vi "Write or Update data Database.vi"(8 "error in (no error)":errorcluster caption="entrée d'erreur (pas d'erreur)", 10 "Function":enum16{"Set Data", "Update Data"}(ring), 11 "Sequencer IN":refnum<class "Sequencer_With_Database.lvclass">) -> (0 "error out":errorcluster caption="sortie d'erreur", 3 "Sequencer Out":refnum<class "Sequencer_With_Database.lvclass">)   [LabVIEW 2020, in "Library Core.lvlib" / "Sequencer_With_Database.lvclass"]
uses:
  Sequencer_With_Database.lvclass
  C:/Users/ngarcin/OneDrive - Altyor/Standard TB/Suite TB45/Class/Sequencer/Sequencer (Default)/Sequencer (Default).lvclass
  Commun VI/TypeDef/Variable Printable.ctl
  Database/Database Altyor/Database Altyor.lvclass
  C:/Users/ngarcin/OneDrive - Altyor/Standard TB/Suite TB45/Class/Database/Database drivers/Database Drivers.lvclass
  JSON API/JSON Value/Set from JSON string.vi
  JSON API/Variant JSON/Variant to JSON.vi
  JSON API/JSON Value/Get Item by name array.vi
  Instrument/Instrument (Default)/Class Instrument (Default).lvclass
  JSON API/JSON Value/JSON Value.lvclass
  Commun VI/Library Commun.lvlib
  JSON API/Variant JSON/Variant JSON.lvlib
  JSON API/Get Polymorphic/JSON GetSet.lvlib
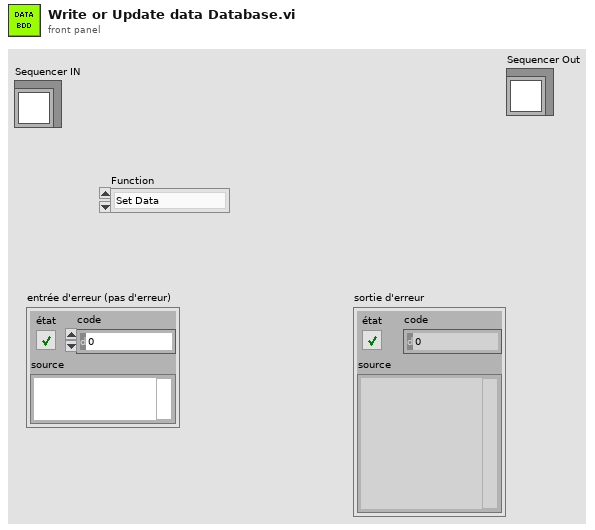
[diagram p1: front panel]
types:
  T1 = cluster{"Connection Name ODBC":string, "DatabaseName":string, "Condition":string, "Type Data ":enum16{"Data Product", "Data Test"}, "Database Altyor":refnum<class "Database Altyor.lvclass">}
  T2 = typedef "Variable Printable.ctl" = string
  T3 = enum16{"Get Variable", "Get All Variables", "Set Variable", "Delete Variable", "Delete All Variable"}
  T4 = cluster{"idTest":u32, "CreationDate":string, "EndOfProduction":string, "OrderNumber":string, "Batch":string, "ProductName":string, "PartNumber":string, "SerialNumber":string, "Operator":string, "Result":string, "AdditionalInformation":string}
  T5 = cluster{"idTest":u32, "CreationDate":string, "EndOfProduction":string, "OrderNumber":string, "Batch":string, "ProductName":string, "PartNumber":string, "SerialNumber":string, "Operator":string, "Result":string, "AdditionalInformation":string}[]
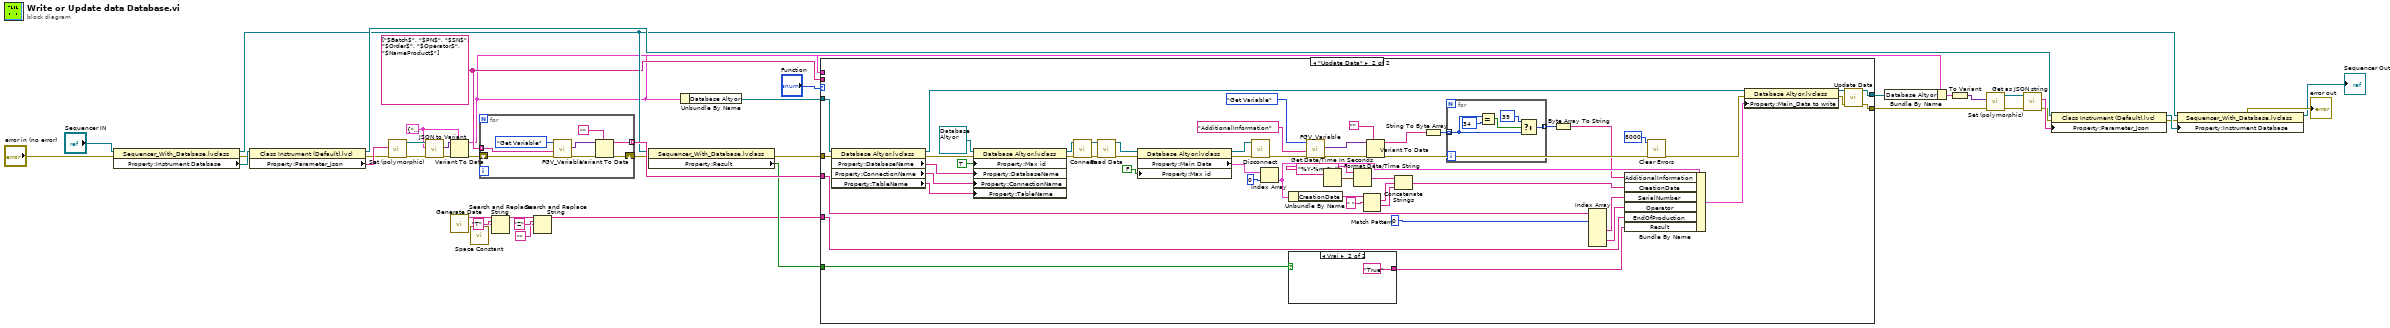
[diagram p0: block diagram]
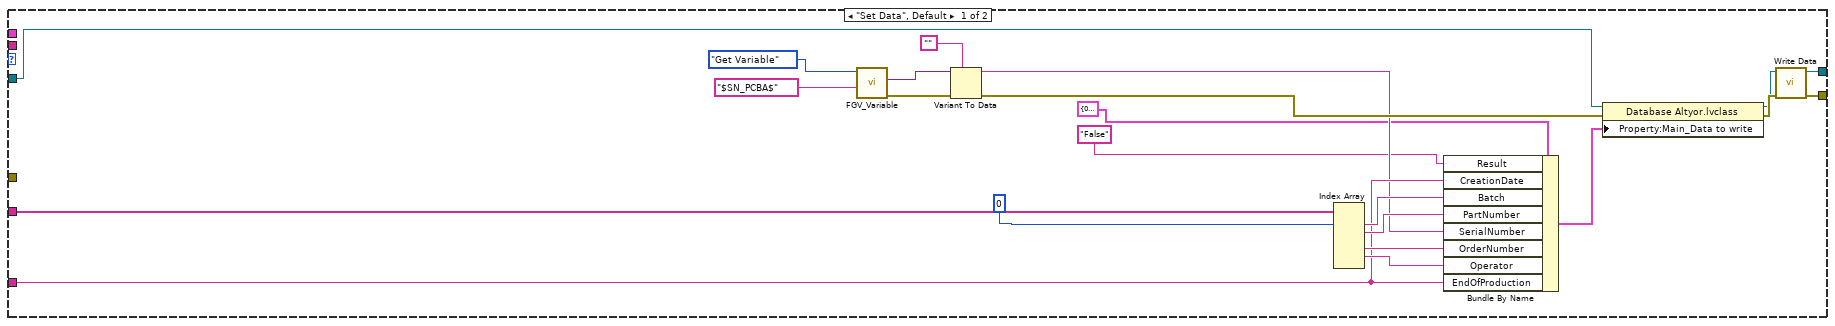
[diagram p2: hidden frame]
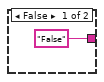
[diagram p3: hidden frame]
diagram:
  w9 = T1 {"Connection Name ODBC"="", "DatabaseName"="", "Condition"="", "Type Data "=enum."Data Product", "Database Altyor"=refnum} ("Parameter")
  w12 = T2[] ["$Batch$", "$PN$", "$SN$", "$Order$", "$Operator$", "$NameProduct$"]
  n1 = property class="Sequencer_With_Database.lvclass"(reference="Sequencer IN", error in="error in (no error)") -> (reference out=w14:refnum<class "Sequencer_With_Database.lvclass">, error out=w39:errorcluster, "Property:Instrument Database"=w40:refnum<class "Class Instrument (Default).lvclass">)
  n2 = property class="Class Instrument (Default).lvcl"(reference=w40, error in=w39) -> (reference out=w24:refnum<class "Class Instrument (Default).lvclass">, error out=w33:errorcluster, "Property:Parameter_Json"=w34:string)
  n3 = call-poly "Set (polymorphic).vi"("error in (no error)"=w33, "JSON stream"=w34) -> ("error out"=w36:errorcluster, "JSON Value out"=w38:refnum<class "JSON Value.lvclass">)  [unwired: 7 in, 1 out]
  n4 = call "JSON to Variant.vi"("error in (no error)"=w36, "Variant (Data Type)"=w9, "JSON Value"=w38) -> ("error out"=w37:errorcluster, "Variant out"=w35:variant)  [unwired: 7 in]
  n5 = Variant To Data(error in=w37, type=w9, Variant=w35) -> (data=w11:T1, error out=w10:errorcluster)
  n6 = call "Generate Date.vi"() -> ("chaîne de date/heure"=w7:string)  [unwired: 11 in]
  n7 = call <vilib>:"Space Constant.vi"() -> ("String"=w5:string)
  n8 = for {
    tunnel: [w46] -> w20 mode=indexing
    shift-right: [w44] -> w19
    shift-left: w10 -> [w43]
    tunnel: w12 -> [w42] mode=indexing
    n9 = call "FGV_Variable.vi"("error in (no error)"=w43, "Variable"=w42, "Function"=T3."Get Variable") -> ("error out"=w45:errorcluster, "Data Out"=w48:variant)  [unwired: 6 in, 1 out]
    n10 = Variant To Data(error in=w45, type="", Variant=w48) -> (data=w46:string, error out=w44:errorcluster)
  }
  n11 = Search and Replace String(input string=w7, search string="T" ("chaîne recherchée"), replace string=w5) -> (result string=w4:string)  [unwired: 5 in, 3 out]
  n12 = Search and Replace String(input string=w4, search string="Z" ("chaîne recherchée"), replace string="") -> (result string=w3:string)  [unwired: 5 in, 3 out]
  n13 = property class="Sequencer_With_Database.lvclass"(reference=w14, error in=w19) -> (error out=w16:errorcluster, "Property:Result"=w15:bool)  [unwired: 1 out]
  n14 = Unbundle By Name(w11) -> ("Database Altyor"=w32:refnum<class "Database Altyor.lvclass">)
  n15 = case shown="\"Update Data\"" "Function" {
    tunnel: [w52 w125] -> w26
    tunnel: w32 -> [w57 w105]
    tunnel: [w50 w124] -> w8
    tunnel: w12 -> [_ _]
    tunnel: w3 -> [w65 w114]
    tunnel: w20 -> [w66 w112]
    tunnel: w16 -> [_ w104]
    tunnel: w15 -> [_ w109]
    tunnel: w11 -> [_ _]
    frame "Set Data", Default {
      n16 = call "FGV_Variable.vi"("Variable"=T2 "$SN_PCBA$", "Function"=T3."Get Variable") -> ("error out"=w61:errorcluster, "Data Out"=w63:variant)  [unwired: 7 in, 1 out]
      n17 = Variant To Data(error in=w61, type="", Variant=w63) -> (data=w58:string, error out=w60:errorcluster)
      n18 = Index Array(array=w66, index #1=0 ("indice")) -> (element #1=w71:string, element #2=w70:string, element #4=w68:string, element #5=w67:string)  [unwired: 5 in, 2 out]
      n19 = Bundle By Name(cluster=T4 {"idTest"=0, "CreationDate"="", "EndOfProduction"="", "OrderNumber"="", "Batch"="", "ProductName"="", "PartNumber"="", "SerialNumber"="", "Operator"="", "Result"="", "AdditionalInformation"=""} ("Main_Data to write"), "Result"="False", "CreationDate"=w65, "Batch"=w71, "PartNumber"=w70, "SerialNumber"=w58, "OrderNumber"=w68, "Operator"=w67, "EndOfProduction"=w65) -> (w54:T4)
      n20 = property class="Database Altyor.lvclass"(reference=w57, error in=w60, "Property:Main_Data to write"=w54) -> (reference out=w51:refnum<class "Database Altyor.lvclass">, error out=w53:errorcluster)
      n21 = call-dynamic "Write Data.vi"("error in (no error)"=w53, "Database Altyor en entrée"=w51) -> ("error out"=w52:errorcluster, "Database Altyor en sortie"=w50:refnum<class "Database Altyor.lvclass">)  [unwired: 8 in]
    }
    frame "Update Data" {
      n22 = property class="Database Altyor.lvclass"(reference=w105, error in=w104) -> (reference out=w96:refnum<class "Database Altyor.lvclass">, error out=w103:errorcluster, "Property:DatabaseName"=w100:string, "Property:ConnectionName"=w99:string, "Property:TableName"=w98:string)
      n23 = property class="Database Altyor.lvclass"(reference=refnum<class "Database Altyor.lvclass"> refnum ("Library Database.lvlib:Database Altyor.lvclass"), error in=w103, "Property:Max id"=TRUE ("Max id"), "Property:DatabaseName"=w100, "Property:ConnectionName"=w99, "Property:TableName"=w98) -> (reference out=w101:refnum<class "Database Altyor.lvclass">, error out=w107:errorcluster)
      n24 = call-dynamic "Connect.vi"("error in (no error)"=w107, "Database Altyor en entrée"=w101) -> ("error out"=w86:errorcluster, "Database Altyor en sortie"=w85:refnum<class "Database Altyor.lvclass">)  [unwired: 8 in]
      n25 = call-dynamic "Read Data.vi"("error in (no error)"=w86, "Database Altyor en entrée"=w85) -> ("error out"=w122:errorcluster, "Database Altyor en sortie"=w123:refnum<class "Database Altyor.lvclass">)  [unwired: 8 in]
      n26 = property class="Database Altyor.lvclass"(reference=w123, error in=w122, "Property:Max id"=FALSE ("Max id")) -> (reference out=w106:refnum<class "Database Altyor.lvclass">, error out=w97:errorcluster, "Property:Main Data"=w120:T5)
      n27 = call-dynamic "Disconnect.vi"("error in (no error)"=w97, "Database Altyor en entrée"=w106) -> ("error out"=w79:errorcluster)  [unwired: 8 in, 1 out]
      n28 = Index Array(array=w120, index=0 ("indice")) -> (element=w95:T4)
      n29 = Unbundle By Name(w95) -> ("CreationDate"=w91:string)
      n30 = case shown="Vrai" w109 {
        tunnel: ["False" "True"] -> w108
        frame False {
        }
        frame True {
        }
      }
      n31 = call "FGV_Variable.vi"("error in (no error)"=w79, "Variable"=T2 "AdditionalInformation", "Function"=T3."Get Variable") -> ("error out"=w82:errorcluster, "Data Out"=w81:variant)  [unwired: 6 in, 1 out]
      n32 = Get Date/Time In Seconds() -> (seconds since 1Jan1904=w93:timestamp)
      n33 = Format Date/Time String(time format string (%c)="%Y-%m-%d" ("chaîne de format de l'heure (%c)"), seconds (now)=w93) -> (date/time string=w89:string)  [unwired: 1 in]
      n34 = Match Pattern(string=w91, regular expression=" " ("expression régulière")) -> (match substring=w90:string, after substring=w88:string)  [unwired: 1 in, 2 out]
      n35 = Variant To Data(error in=w82, type="", Variant=w81) -> (data=w73:string, error out=w78:errorcluster)
      n36 = Concatenate Strings(w89, w90, w88) -> (w87:string)
      n37 = String To Byte Array(string=w73) -> (unsigned byte array=w74:u8[])
      n38 = for {
        tunnel: w74 -> [w127] mode=indexing
        tunnel: [w126] -> w75 mode=indexing
        n39 = Equal?(x=w127, y=u8 34) -> (x = y?=w129:bool)
        n40 = Select(t=u8 39 ("y"), s=w129, f=w127) -> (s? t:f=w126:u8)
      }
      n41 = Byte Array To String(unsigned byte array=w75) -> (string=w72:string)
      n42 = Index Array(array=w112, index #1=0 ("indice")) -> (element #3=w111:string, element #5=w110:string)  [unwired: 5 in, 4 out]
      n43 = Bundle By Name(cluster=w95, "AdditionalInformation"=w72, "CreationDate"=w87, "SerialNumber"=w111, "Operator"=w110, "EndOfProduction"=w114, "Result"=w108) -> (w115:T4)
      n44 = call <vilib>:"Clear Errors.vi"("error in (no error)"=w78, "specific error code to clear (0: all)"=8000) -> ("error out"=w77:errorcluster)  [unwired: 4 in, 1 out]
      n45 = property class="Database Altyor.lvclass"(reference=w96, error in=w77, "Property:Main_Data to write"=w115) -> (reference out=w117:refnum<class "Database Altyor.lvclass">, error out=w118:errorcluster)
      n46 = call-dynamic "Update Data.vi"("error in (no error)"=w118, "Database Altyor en entrée"=w117) -> ("error out"=w125:errorcluster, "Database Altyor en sortie"=w124:refnum<class "Database Altyor.lvclass">)  [unwired: 8 in]
    }
  }
  n47 = Bundle By Name(cluster=w11, "Database Altyor"=w8) -> (w28:T1)
  n48 = To Variant(anything=w28) -> (Variant=w31:variant)
  n49 = call-poly "Set (polymorphic).vi"("error in (no error)"=w26, "Variant"=w31) -> ("error out"=w29:errorcluster, "JSON Value out"=w30:refnum<class "JSON Value.lvclass">)  [unwired: 8 in]
  n50 = call "Get as JSON string.vi"("error in (no error)"=w29, "JSON Value in"=w30) -> ("error out"=w25:errorcluster, "<JSON>"=w27:string)  [unwired: 8 in]
  n51 = property class="Class Instrument (Default).lvcl"(reference=w24, error in=w25, "Property:Parameter_Json"=w27) -> (reference out=w23:refnum<class "Class Instrument (Default).lvclass">, error out=w21:errorcluster)
  n52 = property class="Sequencer_With_Database.lvclass"(reference=w14, error in=w21, "Property:Instrument Database"=w23) -> (reference out=→"Sequencer Out":refnum<class "Sequencer_With_Database.lvclass">, error out=→"error out":errorcluster)
